vi "Spiral Seach.vi"(8 "error in (no error)":errorcluster, 11 "Gantry In":refnum<k24>) -> (0 "error out":errorcluster, 2 "Error?":bool, 3 "Gantry Out":refnum<k24>)   [LabVIEW 2021, in "Component Tray.lvclass"]
uses:
  Component Tray.lvclass
  C:/Program Files (x86)/Aerotech/A3200/LabVIEW/2010/Bin/Aerotech.A3200.dll
  Program Files (x86)/Aerotech/A3200/LabVIEW/2010/Bin/Aerotech.A3200.dll
  Controller/Motion/A3200/A3200.lvclass
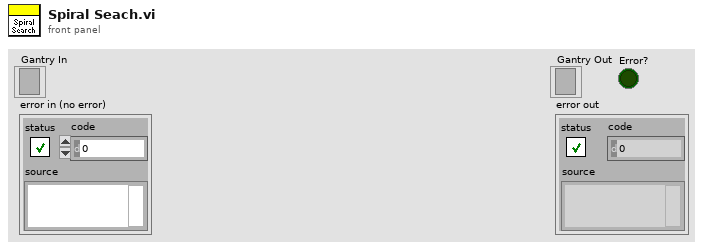
[diagram p1: front panel]
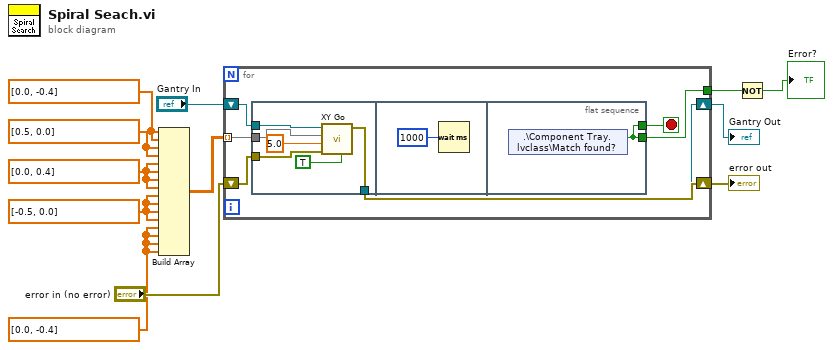
[diagram p0: block diagram]
diagram:
  w3 = dbl[] [0.0, -0.4] ("XY In")
  w4 = dbl[] [-0.5, 0.0] ("XY In")
  w5 = dbl[] [0.0, 0.4] ("XY In")
  w6 = dbl[] [0.5, 0.0] ("XY In")
  w12 = dbl[] [0.0, -0.4] ("XY In")
  n1 = Build Array(w12, w12, w6, w6, w5, w5, w5, w5, w4, w4, w4, w4, w3, w3, w3, w3) -> (w7:dbl[][])
  n2 = for {
    tunnel: w7 -> [w15] mode=indexing
    shift-right: [w17] -> w9
    shift-left: "error in (no error)" -> [w19]
    shift-right: [w16] -> w8
    shift-left: "Gantry In" -> [w18]
    tunnel: [w13] -> w2
    stop <- w14 stop-if-true
    n3 = flat-sequence {
      tunnel: w19 -> [w25]
      tunnel: w18 -> [w23]
      tunnel: [w22] -> w17
      tunnel: [w21] -> w16
      tunnel: w15 -> [w20]
      tunnel: [w28] -> w14
      tunnel: [w28] -> w13
      frame #0 {
        n4 = call "XY Go.vi"("Increment?"=TRUE, "error in (no error)"=w25, "Speed"=5.0, "XY In"=w20, "Gantry In"=w23) -> ("error out"=w22:errorcluster, "Gantry Out"=w21:refnum<k24>)  [unwired: 4 in, 1 out]
      }
      frame #1 {
        n5 = Wait (ms)(milliseconds to wait=u32 1000) -> ()  [unwired: 1 out]
      }
      frame #2 {
        n6 = shared-variable ".\\Component Tray.lvclass\\Match found?"() -> (w28:bool)  [unwired: 1 in, 1 out]
      }
    }
  }
  "Gantry Out" <- w8
  "error out" <- w9
  n7 = Not(x=w2) -> (.not. x?=→"Error?":bool)
